vi "Do.vi"(8 "error in":errorcluster, 10 "Actor in":refnum<class "Actor.lvclass">, 11 "Set TEC Enable MSG":refnum<class "Set TEC Enable MSG.lvclass">) -> (0 "error out":errorcluster, 2 "Actor out":refnum<class "Actor.lvclass">)   [LabVIEW 2014, in "Set TEC Enable MSG.lvclass"]
doc: "(<B>Filename</B>: Actor Framework.lvlib:Message.lvclass:Do.vi)\n\nDefines what a message does when it is received by an actor. Generally, a message instructs an actor to invoke one of its methods. By default, this method does nothing. A child class must override it to define behavior. Create a child class by using the Actor Framework Message Maker dialog box."
uses:
  Set TEC Enable MSG.lvclass
  <vilib>/ActorFramework/Actor/Actor.lvclass
  Set TEC Enable MSG.lvclass/Set TEC Enable MSG.ctl
  Instr Actor.lvclass
  PAS/Commands/Change TEC Enables/Change TEC Enables.lvclass
  PAS/Commands/Change TEC Enables/Change TEC Enables.lvclass/Change TEC Enables.ctl
  Controller/Messages/Update Settings/Children/Array Data/Boolean/Update Bool Array.lvclass
  Controller/Messages/Update Settings/Update Setting.lvclass/Update Setting.ctl
  Controller/Messages/Update Settings/Children/Array Data/Boolean/Update Bool Array.lvclass/Update Bool Array.ctl
  Controller/Messages/Update Settings/Write Key.vi
  Controller/Messages/Update Settings/Children/Array Data/Boolean/Write Setting.vi
  PAS/Commands/Change TEC Enables/Write SP.vi
  reusable/Command/Command.lvclass
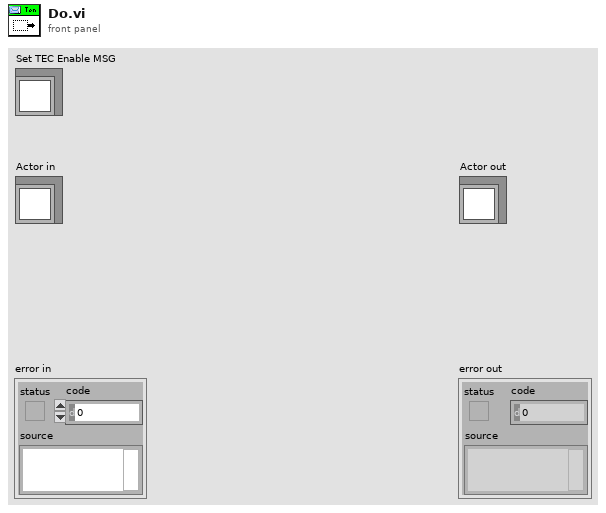
[diagram p1: front panel]
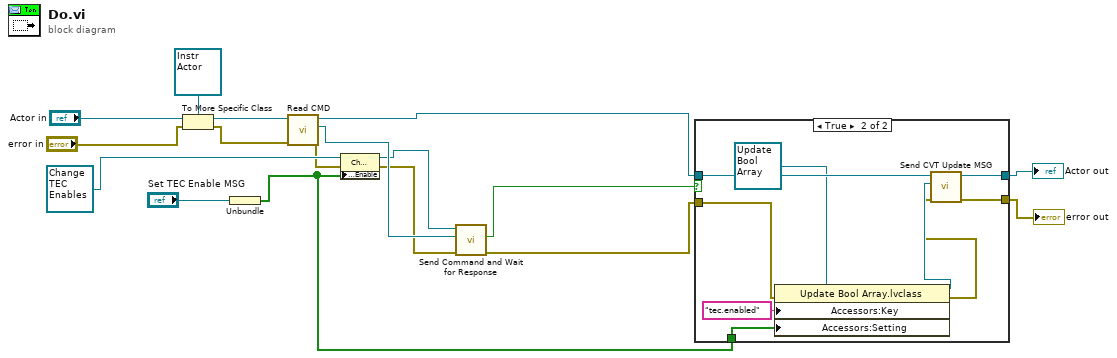
[diagram p0: block diagram]
diagram:
  n1 = To More Specific Class(target class=refnum<class "Instr Actor.lvclass"> refnum ("Instrument Lib:Instr"), reference="Actor in", error in="error in") -> (specific class reference=w15:refnum<class "Instr Actor.lvclass">, error out=w14:errorcluster)
  n2 = Unbundle("Set TEC Enable MSG") -> (w3:bool[])
  n3 = call "Read CMD.vi"("error in (no error)"=w14, "Instr Actor in"=w15) -> ("error out"=w10:errorcluster, "CMD"=w9:refnum<queue>, "Instr Actor out"=w5:refnum<class "Instr Actor.lvclass">)  [unwired: 7 in]
  n4 = property class="Change TEC Enables.lvclass"(reference=refnum<class "Change TEC Enables.lvclass"> refnum ("Change TEC Enables.lvclass"), error in=w10, "Accessors:Enable"=w3) -> (reference out=w8:refnum<class "Change TEC Enables.lvclass">, error out=w7:errorcluster)
  n5 = call "Send Command and Wait for Response.vi"("error in"=w7, "cmd queue"=w9, "CMD in"=w8) -> ("error out"=w2:errorcluster, "cmd good?"=w6:bool)  [unwired: 6 in, 1 out]
  n6 = case shown="True" w6 {
    tunnel: w3 -> [_ w24]
    tunnel: w5 -> [w19 w28]
    tunnel: [w19 w27] -> w4
    tunnel: w2 -> [w18 w22]
    tunnel: [w18 w26] -> w1
    frame False {
    }
    frame True {
      n7 = property class="Update Bool Array.lvclass"(reference=refnum<class "Update Bool Array.lvclass"> refnum ("Controller.lvlib:Update Bool Array.lvclass"), error in=w22, "Accessors:Key"="tec.enabled" ("Key"), "Accessors:Setting"=w24) -> (reference out=w23:refnum<class "Update Bool Array.lvclass">, error out=w21:errorcluster)
      n8 = call "Send CVT Update MSG.vi"("error in (no error)"=w21, "Update Setting"=w23, "Instr in"=w28) -> ("error out"=w26:errorcluster, "Instr out"=w27:refnum<class "Instr Actor.lvclass">)  [unwired: 7 in]
    }
  }
  "error out" <- w1
  "Actor out" <- w4
